vi "DSF.Engine.Memory.Index FIFO.Get FIFO Ref.vi"(8 "error in (no error)":errorcluster, 11 "Index FIFO in":refnum<class "DSF.Engine.Memory.Index FIFO.lvclass">) -> (0 "error out":errorcluster, 2 "FIFO":refnum<k33>, 3 "Index FIFO out":refnum<class "DSF.Engine.Memory.Index FIFO.lvclass">)   [LabVIEW 2016, in "DSF.Engine.lvlib" / "DSF.Engine.Memory.Index FIFO.lvclass"]
uses:
  DSF.Engine.Memory.Index FIFO.lvclass
  DSF.Engine.Memory.Index FIFO.lvclass/DSF.Engine.Memory.Index FIFO.ctl
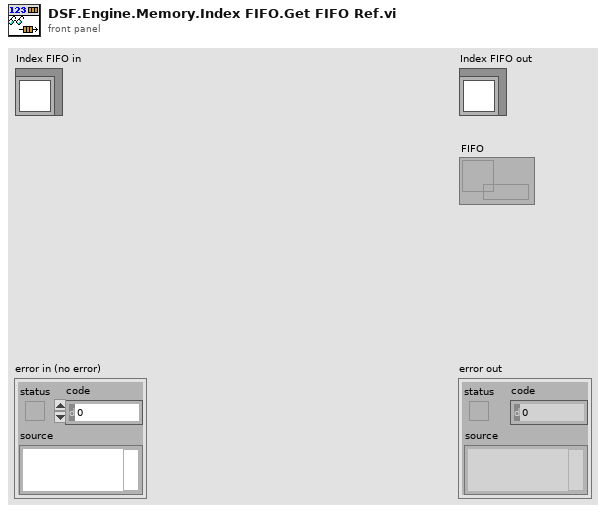
[diagram p1: front panel]
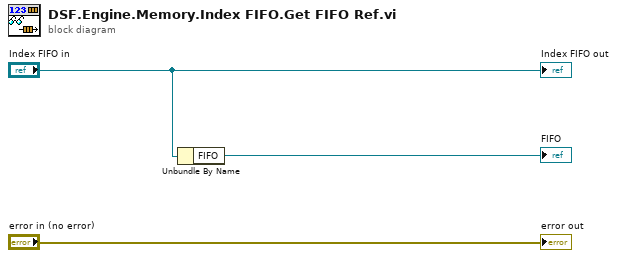
[diagram p0: block diagram]
diagram:
  n1 = Unbundle By Name("Index FIFO in") -> ("FIFO"=→"FIFO":refnum<k33>)
  "error out" <- "error in (no error)"
  "Index FIFO out" <- "Index FIFO in"
